vi "only_wheel.vi"(9 "R_pwm":i32=3000, 10 "L_pwm":i32=3000) -> ()   [LabVIEW 2019]
uses:
  <vilib>/Platform/TimedLoop/XDataNode/timing_clust.ctl
  <vilib>/Platform/TimedLoop/XDataNode/nitl_modes.ctl
  <vilib>/Platform/TimedLoop/XDataNode/wakeup.ctl
  <vilib>/FPGAPlugInAG/myRIO-1900/niLvFpga_Open_myRIO-1900.vi
  <vilib>/rvi/interface/common/dynamic/niFpgaDynamicAddResources.vi
  <vilib>/Utility/error.llb/Error Cluster From Error Code.vi
  <vilib>/rvi/errors/niLvFpgaAdjustHostInterfaceError.vi
  global_stop.vi
  <vilib>/FPGAPlugInAG/Dynamic/niLvFpga_Close_Dynamic.vi
  <vilib>/Platform/TimedLoop/XDataNode/XDataNode.xnode
  <vilib>/rvi/interface/nirviOpenFPGA/nirviOpenFPGA.xnode
  FPGA Bitfiles/capstone_FPGATarget_encoderFPGA_AeXAVEDpCcY.lvbitx
  encoder_FPGA.vi
  <vilib>/rvi/interface/nirviReadWriteControl/nirviReadWriteControl.xnode
  <vilib>/rvi/interface/nirviCloseFPGA/nirviCloseFPGA.xnode
  <vilib>/Platform/TimedLoop/XDataNode/XDNodeRunTimeDep.lvlib
  <vilib>/rvi/interface/Simulation/niFpgaSimulationCallBeginRW.vi
  NiFpgaLv.dll
panel:
  out "회전수":i32
  out "mm/ms":dbl
  out "R_이동 거리":dbl
  out "R_Encoder":i32
  in  "wheel_stop":bool
  out "L_이동 거리":dbl
  out "L_encoder":i32
  out "타임아웃":i32=-1
  out "x > y?":bool
  # "pwm\n3000"
  # "mm/ms\n0.25"
  # "F일 때 앞으로 돌고, T일 때 뒤로 돎"
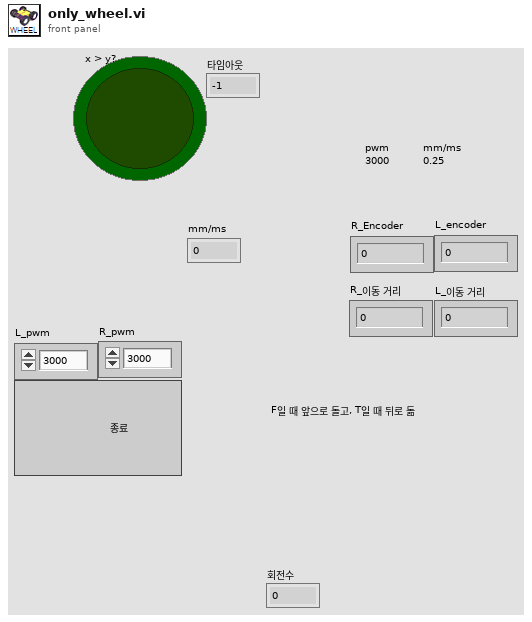
[diagram p1: front panel]
types:
  T1 = typedef "XDNodeRunTimeDep.lvlib/timing_clust.ctl" = cluster{"Expected End [f-1]":u64, "Actual End [f-1]":u64, "Finished Late? [f-1]":bool, "Expected End [i-1]":u64, "Actual End [i-1]":u64, "Finished Late? [i-1]":bool, "Expected Start [i]":u64, "Actual Start [i]":u64, "Expected Start [f]":u64, "Actual Start [f]":u64, "Source Name":string, "Structure Name":string, "Period":i64, "Deadline":i64, "Offset":i64, "Start":i64, "Priority":i32, "Timeout":i32, "Mode":T2, "Wakeup Reason":T3, "Error":errorcluster, "Source Type":string, "Secondary Source Type":string, "Global End Time":u64, "Global Start Time":u64, "Frame Duration":u64, "Iteration Duration":u64, "Assigned CPU":i32, "I/O Scan Engine Mode":u32}
  T2 = typedef "XDNodeRunTimeDep.lvlib/nitl_modes.ctl" = enum32{"No Change", "Process missed periods, maintain original phase", "Discard missed periods, maintain original phase", "Process missed periods, ignore original phase", "Discard missed periods, ignore original phase"}
  T3 = typedef "XDNodeRunTimeDep.lvlib/wakeup.ctl" = enum32{"Normal", "Aborted", "Asynchronous wakeup", "Timing source error", "Timed loop error", "Timeout"}
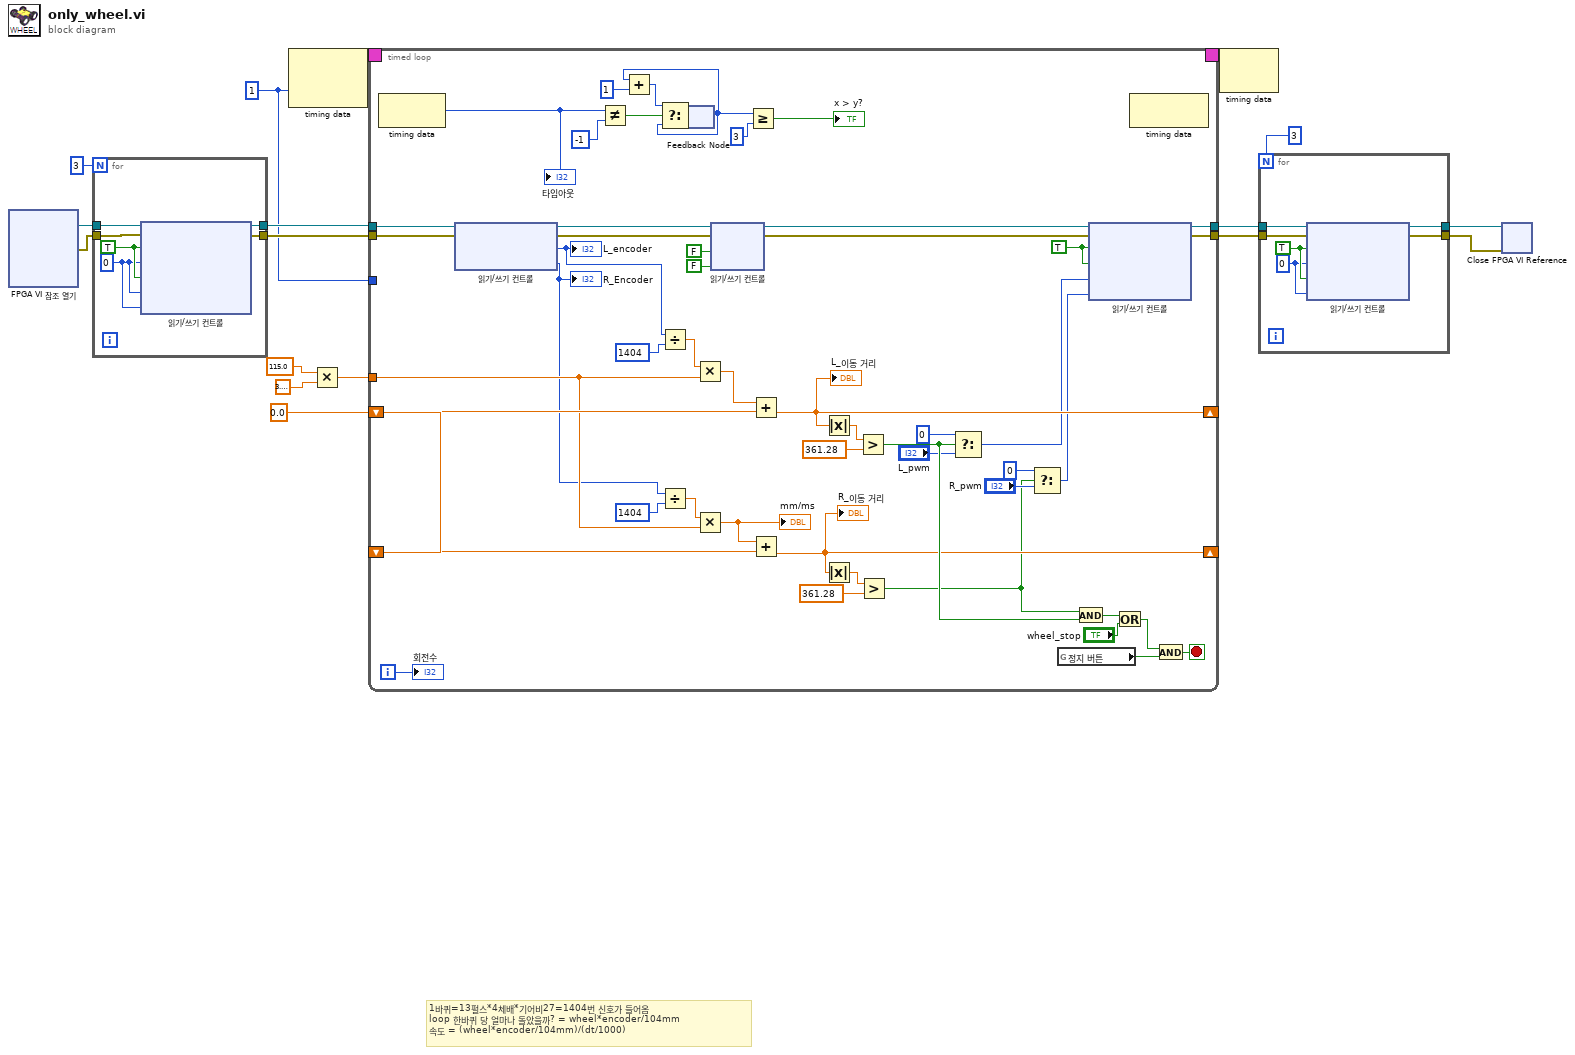
[diagram p0: block diagram]
diagram:
  w5 = 0.0
  w6 = i64 1 ("주기")
  # "1바퀴=13펄스*4체배*기어비27=1404번 신호가 들어옴\nloop 한바퀴 당 얼마나 돌았을까? = wheel*encoder/104mm\n속도 = (wheel*encoder/104mm)/(dt/1000)"
  n1 = xnode "FPGA VI 참조 열기"() -> ("FPGA VI 참조 출력"=w4:refnum<k20>, "에러 출력"=w3:errorcluster)  [unwired: 2 in]
  n2 = for {
    N: 3 -> [_]
    tunnel: [w23] -> w14
    tunnel: [w22] -> w13
    tunnel: w4 -> [w19]
    tunnel: w3 -> [w18]
    w20 = 0 ("pwm input(escon)")
    w21 = TRUE ("encoder reset")
    n3 = xnode "읽기/쓰기 컨트롤"("FPGA VI 참조 입력"=w19, "에러 입력"=w18, "encoder reset"=w21, "pwm input"=w20, "R_encoder reset"=w21, "R_pwm input"=w20, "직동_pwm input"=w20) -> ("FPGA VI 참조 출력"=w23:refnum<k20>, "에러 출력"=w22:errorcluster)
  }
  n4 = node-c288(w6) -> (w17:T1)  [unwired: 1 in]
  n5 = Multiply(x=115.0, y=3.141592653589793) -> (x*y=w7:dbl)
  n6 = timed-loop {
    timing: w17 -> [_]
    timing-out: [_] -> w16
    tunnel: w14 -> [w62]
    tunnel: w13 -> [w61]
    tunnel: [w65] -> w12
    tunnel: [w64] -> w11
    tunnel: w7 -> [w53]
    tunnel: w6 -> [_]
    shift-right: [w56] -> _
    shift-left: w5 -> [w54]
    shift-right: [w26] -> _
    shift-left: w5 -> [w55]
    i -> [w24]
    stop <- w36 stop-if-true
    w63 = TRUE ("encoder reset")
    n7 = node-c288() -> (w74:i32)  [unwired: 1 in]
    "타임아웃" <- w74
    n8 = xnode "읽기/쓰기 컨트롤"("FPGA VI 참조 입력"=w62, "에러 입력"=w61) -> ("FPGA VI 참조 출력"=w59:refnum<k20>, "에러 출력"=w58:errorcluster, "Encoder  (4x)"=w52:i32, "R_Encoder  (4x)"=w51:i32)
    "L_encoder" <- w52
    "R_Encoder" <- w51
    n9 = Not Equal?(x=w74, y=-1) -> (x != y?=w72:bool)
    n10 = Divide(x=w52, y=1404) -> (x/y=w45:dbl)
    n11 = Divide(x=w51, y=1404) -> (x/y=w40:dbl)
    n12 = feedback #1() -> (w68:u8)  [unwired: 1 in]
    n13 = Add(x=w68, y=u8 1) -> (x+y=w71:u8)
    n14 = Select(t=w71, s=w72, f=w68) -> (s? t:f=w70:u8)
    n15 = feedback-in #1(w70) -> ()
    n16 = Multiply(x=w45, y=w53) -> (x*y=w47:dbl)
    n17 = Multiply(x=w40, y=w53) -> (x*y=w42:dbl)
    "mm/ms" <- w42
    n18 = xnode "읽기/쓰기 컨트롤"("FPGA VI 참조 입력"=w59, "에러 입력"=w58, "R_dir"=FALSE, "L_dir"=FALSE) -> ("FPGA VI 참조 출력"=w60:refnum<k20>, "에러 출력"=w57:errorcluster)
    n19 = Greater Or Equal?(x=w68, y=u8 3) -> (x >= y?=→"x > y?":bool)
    n20 = Add(x=w47, y=w54) -> (x+y=w56:dbl)
    "L_이동 거리" <- w56
    n21 = Add(x=w42, y=w55) -> (x+y=w26:dbl)
    "R_이동 거리" <- w26
    n22 = Absolute Value(x=w56) -> (abs(x)=w44:dbl)
    n23 = Absolute Value(x=w26) -> (abs(x)=w39:dbl)
    n24 = Greater?(x=w44, y=361.28) -> (0:w33:bool)
    n25 = Greater?(x=w39, y=361.28) -> (0:w25:bool)
    n26 = Select(t=0, s=w33, f="L_pwm") -> (s? t:f=w32:i32)
    n27 = Select(t=0, s=w25, f="R_pwm") -> (s? t:f=w27:i32)
    n28 = global read "global_stop.vi" "정지 버튼"() -> (w35:bool)
    n29 = And(x=w25, y=w33) -> (x .and. y?=w38:bool)
    n30 = xnode "읽기/쓰기 컨트롤"("FPGA VI 참조 입력"=w60, "에러 입력"=w57, "encoder reset"=w63, "R_encoder reset"=w63, "pwm input"=w32, "R_pwm input"=w27) -> ("FPGA VI 참조 출력"=w65:refnum<k20>, "에러 출력"=w64:errorcluster)
    n31 = Or(x=w38, y="wheel_stop") -> (x .or. y?=w34:bool)
    n32 = node-c288() -> ()  [unwired: 1 in, 1 out]
    n33 = And(x=w34, y=w35) -> (x .and. y?=w36:bool)
    "회전수" <- w24
  }
  n34 = node-c288(w16) -> ()  [unwired: 1 out]
  n35 = for {
    N: 3 -> [_]
    tunnel: w12 -> [w83]
    tunnel: w11 -> [w82]
    tunnel: [w79] -> w2
    tunnel: [w78] -> w1
    w80 = 0 ("pwm input(escon)")
    w81 = TRUE ("encoder reset")
    n36 = xnode "읽기/쓰기 컨트롤"("FPGA VI 참조 입력"=w83, "에러 입력"=w82, "encoder reset"=w81, "pwm input"=w80, "R_encoder reset"=w81, "R_pwm input"=w80) -> ("FPGA VI 참조 출력"=w79:refnum<k20>, "에러 출력"=w78:errorcluster)
  }
  n37 = xnode "Close FPGA VI Reference"("FPGA VI 참조 입력"=w2, "에러 입력"=w1) -> ()  [unwired: 1 out]
